vi "example test.vi"() -> ()   [LabVIEW 2013, in "TEC tests.lvlib"]
uses:
  TEC tests.lvlib
  configuration/TEC configuration.lvclass
  execution/TEC runtime.lvclass
  <vilib>/NI/Tag Bus/tag/Data Type.ctl
  <vilib>/NI/Tag Bus Module Framework/channel/channel classification.ctl
  configuration/TEC configuration.lvclass/TEC configuration.ctl
  <vilib>/NI/Tag Bus/table/data polymorphs/write one/write Double.vi
  <vilib>/NI/Tag Bus/table/data polymorphs/read one/read Double.vi
  configuration/Write receive on port.vi
  configuration/Write send from port.vi
  configuration/Write send to address.vi
  configuration/Write send to port.vi
  <vilib>/NI/Tag Bus Module Framework/channel/TBM channel.lvclass
  <vilib>/NI/Tag Bus/tag/tag descriptor.lvclass
  <vilib>/NI/Tag Bus/table/data table.lvlib
  <vilib>/ptbypt/NI_PtbyPt.lvlib
panel:
  out "duration avg":dbl
  in  "millisecond multiple":u32=100
  out "duration":dbl
  out "timeout count":u16
  out "final":errorcluster
  out "value rx":dbl
  in  "value tx":dbl
  in  "stop":bool
  out "init err":errorcluster
  in  "ch count":i32=100
  out "serialization problem":errorcluster
  out "invalid configuration":errorcluster
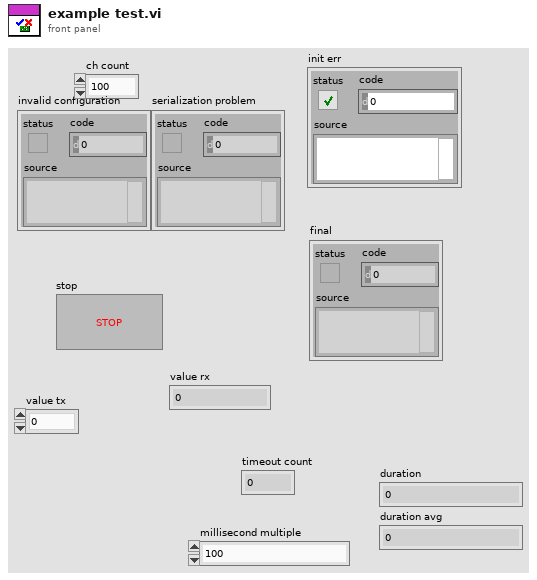
[diagram p1: front panel]
types:
  T1 = typedef "TBM channel.lvclass/channel classification.ctl" = enum16{"input data", "output data", "processing parameter", "processing result"}
  T2 = typedef "tag bus.lvlib/tag descriptor.lvclass/Data Type.ctl" = enum16{"Double", "Single", "I64", "I32", "I16", "I8", "U64", "U32", "U16", "U8", "Boolean", "String", "Array of Double", "Array of Single", "Array of I64", "Array of I32", "Array of I16", "Array of I8", "Array of U64", "Array of U32", "Array of U16", "Array of U8", "Array of Boolean", "Array of String"}
  T3 = typedef "TBM channel.lvclass/data tables.ctl" = cluster{"input data":T4, "processing parameter":T4, "processing result":T4, "output data":T4}
  T4 = typedef "tag bus.lvlib/dictionary table pair.ctl" = cluster{"data dictionary":refnum<class "data dictionary.lvclass">, "data table":T5}
  T5 = typedef "tag bus.lvlib/data table.lvlib/data table.ctl" = cluster{"Double":dbl[], "Single":sgl[], "I64":i64[], "I32":i32[], "I16":i16[], "I8":i8[], "U64":u64[], "U32":u32[], "U16":u16[], "U8":u8[], "Boolean":bool[], "String":string[], "Array of Double":cluster{"DBL Array":dbl[]}[], "Array of Single":cluster{"SGL Array":sgl[]}[], "Array of I64":cluster{"I64 Array":i64[]}[], "Array of I32":cluster{"I32 Array":i32[]}[], "Array of I16":cluster{"I16 Array":i16[]}[], "Array of I8":cluster{"I8 Array":i8[]}[], "Array of U64":cluster{"U64 Array":u64[]}[], "Array of U32":cluster{"U32 Array":u32[]}[], "Array of U16":cluster{"U16 Array":u16[]}[], "Array of U8":cluster{"U8 Array":u8[]}[], "Array of Boolean":cluster{"Boolean Array":bool[]}[], "Array of String":cluster{"String Array":string[]}[]}
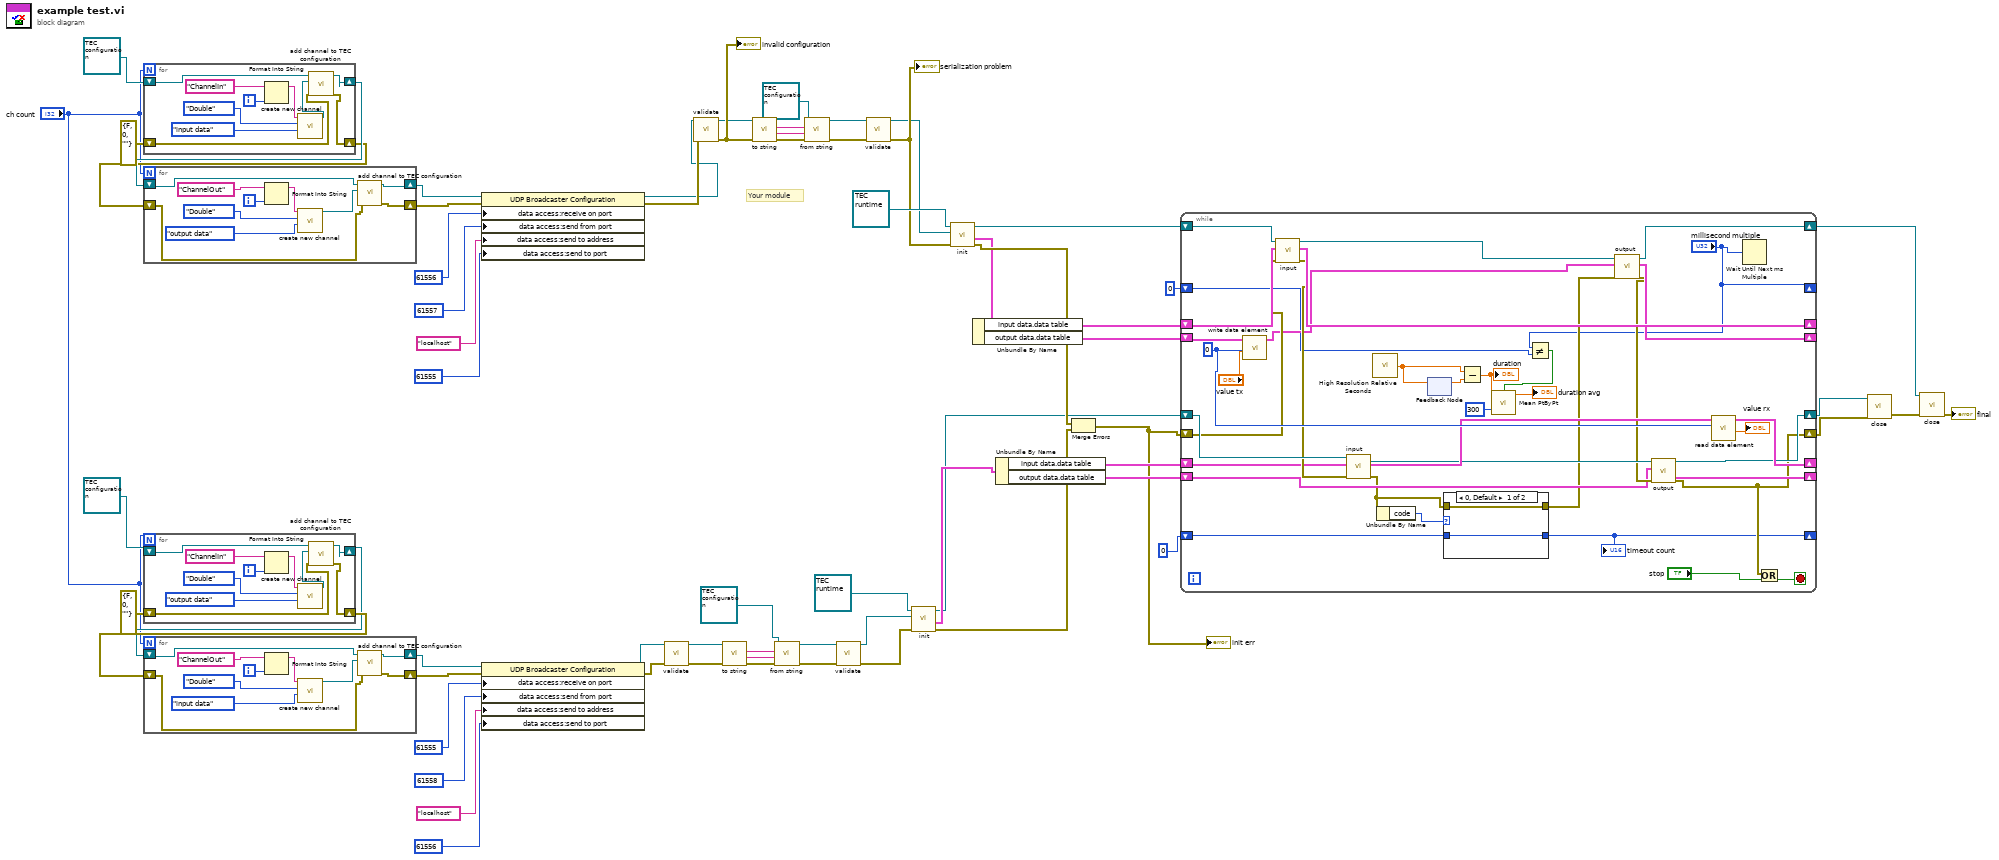
[diagram p0: block diagram]
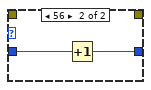
[diagram p2: hidden frame]
diagram:
  # "Your module"
  n1 = for {
    N: "ch count" -> [_]
    shift-right: [w69] -> w55
    shift-left: refnum<class "TEC configuration.lvclass"> refnum ("tag bus configurable plugin module configuration") -> [w68]
    shift-right: [w70] -> w53
    shift-left: errorcluster {"status"=FALSE, "code"=0, "source"=""} ("error out") -> [w66]
    i -> [w73]
    n2 = Format Into String(initial string="ChannelIn" ("channel name"), w73) -> (resulting string=w72:string)  [unwired: 2 in, 1 out]
    n3 = call <vilib>:"create new channel.vi"("channel classification"=channel_classification."input data", "data type"=Data_Type."Double", "channel name"=w72) -> ("channel"=w67:refnum<class "TBM channel.lvclass">)  [unwired: 8 in]
    n4 = call "add channel to TEC configuration.vi"("error in"=w66, "channel"=w67, "TEC configuration in"=w68) -> ("error out"=w70:errorcluster, "TEC configuration out"=w69:refnum<class "TEC configuration.lvclass">)  [unwired: 7 in]
  }
  n5 = for {
    N: "ch count" -> [_]
    shift-right: [w77] -> w50
    shift-left: w55 -> [w80]
    shift-right: [w78] -> w54
    shift-left: w53 -> [w79]
    i -> [w83]
    n6 = Format Into String(initial string="ChannelOut" ("channel name"), w83) -> (resulting string=w82:string)  [unwired: 2 in, 1 out]
    n7 = call <vilib>:"create new channel.vi"("channel classification"=channel_classification."output data", "data type"=Data_Type."Double", "channel name"=w82) -> ("channel"=w76:refnum<class "TBM channel.lvclass">)  [unwired: 8 in]
    n8 = call "add channel to TEC configuration.vi"("error in"=w79, "channel"=w76, "TEC configuration in"=w80) -> ("error out"=w78:errorcluster, "TEC configuration out"=w77:refnum<class "TEC configuration.lvclass">)  [unwired: 7 in]
  }
  n9 = for {
    N: "ch count" -> [_]
    shift-right: [w89] -> w36
    shift-left: refnum<class "TEC configuration.lvclass"> refnum ("tag bus configurable plugin module configuration") -> [w88]
    shift-right: [w90] -> w38
    shift-left: errorcluster {"status"=FALSE, "code"=0, "source"=""} ("error out") -> [w86]
    i -> [w93]
    n10 = Format Into String(initial string="ChannelIn" ("channel name"), w93) -> (resulting string=w92:string)  [unwired: 2 in, 1 out]
    n11 = call <vilib>:"create new channel.vi"("channel classification"=channel_classification."output data", "data type"=Data_Type."Double", "channel name"=w92) -> ("channel"=w87:refnum<class "TBM channel.lvclass">)  [unwired: 8 in]
    n12 = call "add channel to TEC configuration.vi"("error in"=w86, "channel"=w87, "TEC configuration in"=w88) -> ("error out"=w90:errorcluster, "TEC configuration out"=w89:refnum<class "TEC configuration.lvclass">)  [unwired: 7 in]
  }
  n13 = for {
    N: "ch count" -> [_]
    shift-right: [w97] -> w40
    shift-left: w36 -> [w100]
    shift-right: [w98] -> w37
    shift-left: w38 -> [w99]
    i -> [w103]
    n14 = Format Into String(initial string="ChannelOut" ("channel name"), w103) -> (resulting string=w102:string)  [unwired: 2 in, 1 out]
    n15 = call <vilib>:"create new channel.vi"("channel classification"=channel_classification."input data", "data type"=Data_Type."Double", "channel name"=w102) -> ("channel"=w96:refnum<class "TBM channel.lvclass">)  [unwired: 8 in]
    n16 = call "add channel to TEC configuration.vi"("error in"=w99, "channel"=w96, "TEC configuration in"=w100) -> ("error out"=w98:errorcluster, "TEC configuration out"=w97:refnum<class "TEC configuration.lvclass">)  [unwired: 7 in]
  }
  n17 = property class="UDP Broadcaster Configuration"(reference=w50, error in=w54, "data access:receive on port"=u16 61556 ("send from port"), "data access:send from port"=u16 61557 ("send to port"), "data access:send to address"="localhost" ("send to address"), "data access:send to port"=u16 61555 ("receive on port")) -> (reference out=w49:refnum<class "TEC configuration.lvclass">, error out=w51:errorcluster)
  n18 = property class="UDP Broadcaster Configuration"(reference=w40, error in=w37, "data access:receive on port"=u16 61555 ("send from port"), "data access:send from port"=u16 61558 ("send to port"), "data access:send to address"="localhost" ("send to address"), "data access:send to port"=u16 61556 ("receive on port")) -> (reference out=w23:refnum<class "TEC configuration.lvclass">, error out=w24:errorcluster)
  n19 = call-dynamic "validate.vi"("error in"=w24, "TEC configuration in"=w23) -> ("error out"=w25:errorcluster, "TEC configuration out"=w31:refnum<class "TEC configuration.lvclass">)  [unwired: 8 in]
  n20 = call-dynamic "validate.vi"("error in"=w51, "TEC configuration in"=w49) -> ("error out"=w65:errorcluster, "TEC configuration out"=w33:refnum<class "TEC configuration.lvclass">)  [unwired: 8 in]
  "invalid configuration" <- w65
  n21 = call-dynamic "to string.vi"("error in"=w25, "TEC configuration in"=w31) -> ("error out"=w28:errorcluster, "data"=w27:string, "version"=w26:string)  [unwired: 6 in, 1 out]
  n22 = call-dynamic "to string.vi"("error in"=w65, "TEC configuration in"=w33) -> ("error out"=w62:errorcluster, "data"=w63:string, "version"=w64:string)  [unwired: 6 in, 1 out]
  n23 = call-dynamic "from string.vi"("error in"=w28, "data"=w27, "version"=w26, "TEC configuration in"=refnum<class "TEC configuration.lvclass"> refnum) -> ("error out"=w30:errorcluster, "TEC configuration out"=w29:refnum<class "TEC configuration.lvclass">)  [unwired: 6 in]
  n24 = call-dynamic "from string.vi"("error in"=w62, "data"=w63, "version"=w64, "TEC configuration in"=refnum<class "TEC configuration.lvclass"> refnum) -> ("error out"=w60:errorcluster, "TEC configuration out"=w61:refnum<class "TEC configuration.lvclass">)  [unwired: 6 in]
  n25 = call-dynamic "validate.vi"("error in"=w30, "TEC configuration in"=w29) -> ("error out"=w21:errorcluster, "TEC configuration out"=w20:refnum<class "TEC configuration.lvclass">)  [unwired: 8 in]
  n26 = call-dynamic "validate.vi"("error in"=w60, "TEC configuration in"=w61) -> ("error out"=w58:errorcluster, "TEC configuration out"=w57:refnum<class "TEC configuration.lvclass">)  [unwired: 8 in]
  "serialization problem" <- w58
  n27 = call-dynamic "init.vi"("error in"=w21, "TBM module configuration in"=w20, "TEC runtime in"=refnum<class "TEC runtime.lvclass"> refnum ("tag bus configurable plugin module")) -> ("error out"=w18:errorcluster, "data allocations"=w15:T3, "TEC runtime out"=w9:refnum<class "TEC runtime.lvclass">)  [unwired: 5 in, 1 out]
  n28 = call-dynamic "init.vi"("error in"=w58, "TBM module configuration in"=w57, "TEC runtime in"=refnum<class "TEC runtime.lvclass"> refnum ("tag bus configurable plugin module")) -> ("error out"=w19:errorcluster, "data allocations"=w16:T3, "TEC runtime out"=w10:refnum<class "TEC runtime.lvclass">)  [unwired: 5 in, 1 out]
  n29 = Unbundle By Name(w16) -> ("input data.data table"=w12:T5, "output data.data table"=w11:T5)
  n30 = Unbundle By Name(w15) -> ("input data.data table"=w14:T5, "output data.data table"=w13:T5)
  n31 = Merge Errors(w19, w18) -> (w8:errorcluster)
  "init err" <- w8
  n32 = while {
    shift-right: [w139] -> _
    shift-left: w14 -> [w130]
    shift-right: [w122] -> _
    shift-left: w13 -> [w119]
    shift-right: [w125] -> _
    shift-left: w11 -> [w141]
    shift-right: [w134] -> _
    shift-left: w12 -> [w135]
    shift-right: [w127] -> w4
    shift-left: w10 -> [w136]
    shift-right: [w123] -> w3
    shift-left: w9 -> [w133]
    shift-right: [w120] -> w7
    shift-left: w8 -> [w132]
    shift-right: [w115] -> _
    shift-left: u16 0 ("Numeric") -> [w114]
    shift-right: ["millisecond multiple"] -> _
    shift-left: u32 0 ("millisecond multiple") -> [w108]
    stop <- w142 stop-if-true
    w137 = 0 ("index")
    n33 = call-poly <vilib>:"write data element.vi"("value"="value tx", "index"=w137, "data table in"=w141) -> ("data table out"=w126:T5)  [unwired: 8 in]
    n34 = call-dynamic "input.vi"("error in"=w132, "data table in"=w135, "TEC runtime in"=w136) -> ("error out"=w131:errorcluster, "data table out"=w134:T5, "TEC runtime out"=w128:refnum<class "TEC runtime.lvclass">)  [unwired: 6 in]
    n35 = call-dynamic "input.vi"("error in"=w131, "data table in"=w130, "TEC runtime in"=w133) -> ("error out"=w117:errorcluster, "data table out"=w129:T5, "TEC runtime out"=w124:refnum<class "TEC runtime.lvclass">)  [unwired: 6 in]
    n36 = call <vilib>:"High Resolution Relative Seconds.vi"() -> ("relative seconds"=w112:dbl)
    n37 = Unbundle By Name(w117) -> ("code"=w118:i32)
    n38 = feedback-in #1(w112) -> ()
    n39 = feedback #1() -> (w113:dbl)  [unwired: 1 in]
    n40 = case shown="0, Default" w118 {
      tunnel: w117 -> [w145 _]
      tunnel: [w145 _] -> w116
      tunnel: [w144 w147] -> w115
      tunnel: w114 -> [w144 w146]
      frame 0, Default {
      }
      frame 56 {
        n41 = Increment(x=w146) -> (x+1=w147:u16)
      }
    }
    "timeout count" <- w115
    n42 = Subtract(x=w112, y=w113) -> (x-y=w111:dbl)
    "duration" <- w111
    n43 = Not Equal?(x="millisecond multiple", y=w108) -> (x != y?=w107:bool)
    n44 = call <vilib>:"Mean PtByPt.vi"("x"=w111, "sample length"=300, "initialize"=w107) -> ("mean"=→"duration avg":dbl)  [unwired: 1 in, 1 out]
    n45 = call-dynamic "output.vi"("error in"=w116, "data table in"=w126, "TEC runtime in"=w128) -> ("error out"=w121:errorcluster, "data table out"=w125:T5, "TEC runtime out"=w127:refnum<class "TEC runtime.lvclass">)  [unwired: 6 in]
    n46 = call-dynamic "output.vi"("error in"=w121, "data table in"=w119, "TEC runtime in"=w124) -> ("error out"=w120:errorcluster, "data table out"=w122:T5, "TEC runtime out"=w123:refnum<class "TEC runtime.lvclass">)  [unwired: 6 in]
    n47 = call-poly <vilib>:"read data element.vi"("index"=w137, "data table in"=w129) -> ("value"=→"value rx":dbl, "data table out"=w139:T5)  [unwired: 8 in]
    n48 = Wait Until Next ms Multiple(millisecond multiple="millisecond multiple") -> ()  [unwired: 1 out]
    n49 = Or(x=w120, y="stop") -> (x .or. y?=w142:bool)
  }
  n50 = call-dynamic "close.vi"("error in"=w7, "TEC runtime in"=w3) -> ("error out"=w6:errorcluster)  [unwired: 9 in]
  n51 = call-dynamic "close.vi"("error in"=w6, "TEC runtime in"=w4) -> ("error out"=→"final":errorcluster)  [unwired: 9 in]
